vi "Initialize.vi"(8 "error in":errorcluster, 11 "Ballard MIL-STD-1553 custom device in":T1 format="%.0x") -> (0 "error out":errorcluster, 3 "Ballard MIL-STD-1553 custom device out":T1 format="%.0x")   [LabVIEW 2020, in "Ballard MIL-STD-1553 System Explorer.lvlib" / "Implementation.lvlib"]
uses:
  Implementation.lvlib
  <vilib>/NI VeriStand/Custom Device API/Custom Device Item Ref.ctl
  Shared/Device Parameters.ctl
  Shared/Initialization Method.ctl
  Scripting/Ballard MIL-STD-1553 Scripting.lvlib
  <vilib>/NI VeriStand/Custom Device API/Custom Device API.lvlib
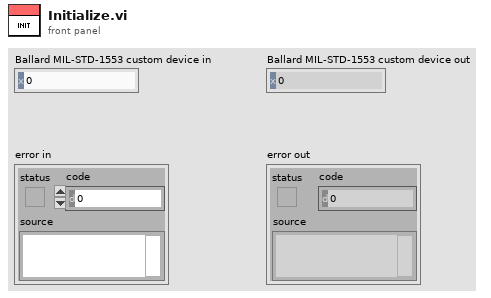
[diagram p1: front panel]
types:
  T1 = typedef "Custom Device API.lvlib/Custom Device Item Ref.ctl" = u64
  T2 = typedef "Device Parameters.ctl" = cluster{"initialization method":T3, "card number":i32, "PXI slot number":i32, "core number":i32}
  T3 = typedef "Initialization Method.ctl" = enum16{"PXI Slot Number", "Card Number"}
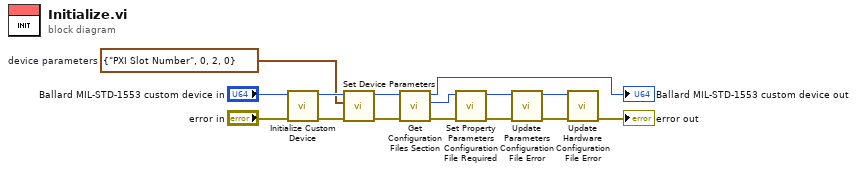
[diagram p0: block diagram]
diagram:
  w11 = T2 {"initialization method"=enum."PXI Slot Number", "card number"=0, "PXI slot number"=2, "core number"=0}  # device parameters
  n1 = call "Initialize Custom Device.vi"("error in"="error in", "Ballard MIL-STD 1553 in"="Ballard MIL-STD-1553 custom device in") -> ("error out"=w13:errorcluster, "Ballard MIL-STD 1553 out"=w12:T1)  [unwired: 8 in]
  n2 = call "Set Device Parameters.vi"("error in"=w13, "device parameters"=w11, "Ballard MIL-STD 1553 custom device in"=w12) -> ("error out"=w9:errorcluster, "Ballard MIL-STD 1553 custom device out"=w10:T1)  [unwired: 7 in]
  n3 = call "Get Configuration Files Section.vi"("error in"=w9, "custom device in"=w10) -> ("error out"=w6:errorcluster, "configuration files section"=w7:T1, "custom device out"=→"Ballard MIL-STD-1553 custom device out":T1)  [unwired: 7 in]
  n4 = call "Set Property Parameters Configuration File Required.vi"("error in"=w6, "configuration files ref"=w7) -> ("error out"=w4:errorcluster, "configuration files ref out"=w5:T1)  [unwired: 8 in]
  n5 = call "Update Parameters Configuration File Error.vi"("error in"=w4, "configuration files ref in"=w5) -> ("error out"=w2:errorcluster, "configuration files ref out"=w3:T1)  [unwired: 8 in]
  n6 = call "Update Hardware Configuration File Error.vi"("error in"=w2, "configuration files ref in"=w3) -> ("error out"=→"error out":errorcluster)  [unwired: 8 in, 1 out]
